vi "Remove Topic Subscriber.vi"(8 "error in (no error)":errorcluster, 10 "Unique Subscriber ID":string, 11 "Topic in":refnum<class "Topic.lvclass">) -> (0 "error out":errorcluster, 3 "Topic out":refnum<class "Topic.lvclass">)   [LabVIEW 2015, in "Mediator.lvlib" / "Topic.lvclass"]
doc: "<License>\nCopyright © 2017 Composed Systems, LLC | All rights reserved\nwww.composed.io\n\nAuthor: Ethan Stern <ethan.stern@composed.io>\n\nThis software is provided \"AS IS\" WITHOUT WARRANTIES, either express or implied, AND IS FOR EDUCATIONAL PURPOSES ONLY.\n</License>"
uses:
  Topic.lvclass
  Topic.lvclass/Topic.ctl
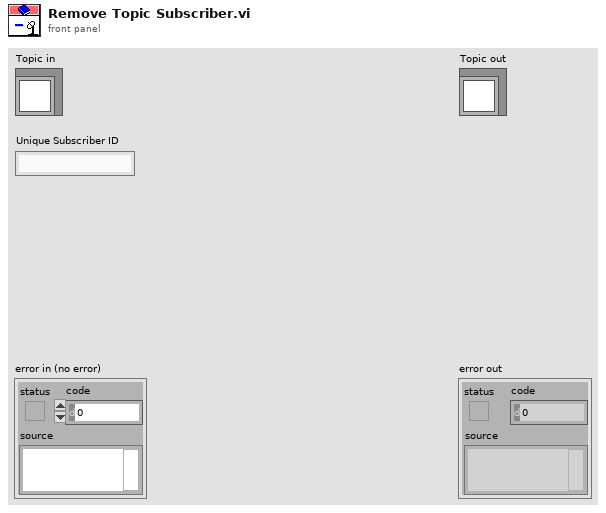
[diagram p1: front panel]
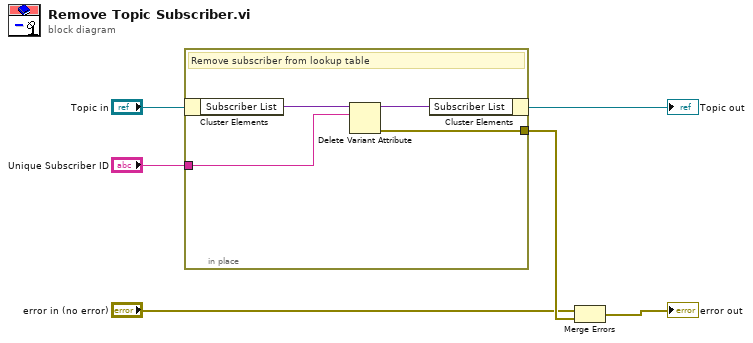
[diagram p0: block diagram]
diagram:
  n1 = in-place {
    in-place-border: [w9] -> w6
    in-place-border: "Unique Subscriber ID" -> [w8]
    # "Remove subscriber from lookup table"
    n2 = in-place-cluster #1("Topic in") -> ("Subscriber List"=w7:variant)
    n3 = Delete Variant Attribute(6:w8, 7:w7) -> (0:w9:errorcluster, 3:w10:variant)  [unwired: 1 in, 1 out]
    n4 = in-place-cluster #1("Subscriber List"=w10) -> (→"Topic out":refnum<class "Topic.lvclass">)
  }
  n5 = Merge Errors("error in (no error)", w6) -> (→"error out":errorcluster)
